vi "Update Status.vi"(9 "Spec Page Interface":T1, 11 "ADAS_IO_Template_MDO.lvclass":refnum<class "ADAS_IO_Template_MDO.lvclass">) -> ()   [LabVIEW 2020, in "ADAS_IO_Template_MDO.lvclass"]
uses:
  ADAS_IO_Template_MDO.lvclass
  <resource>/dialog/NewProjectWizard/Spec Page Interface.ctl
  ADAS_IO_Template_MDO.lvclass/ADAS_IO_Template_MDO.ctl
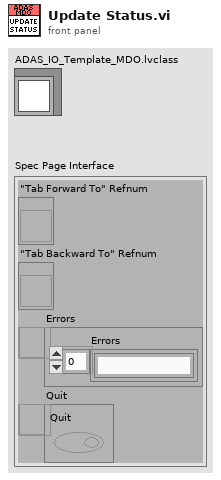
[diagram p1: front panel]
types:
  T1 = typedef "Spec Page Interface.ctl" = cluster{"\"Tab Forward To\" Refnum":refnum<vi>, "\"Tab Backward To\" Refnum":refnum<vi>, "Errors":refnum<user-event>, "Quit":refnum<user-event>}
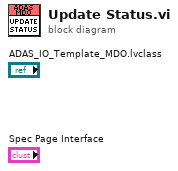
[diagram p0: block diagram]
diagram:
